vi "simx Get Joint Position.vi"(7 "operationMode":i32, 8 "error in (no error)":errorcluster, 9 "position":sgl, 10 "jointHandle":i32, 11 "clientID":i32) -> (0 "error out":errorcluster, 1 "position out":sgl, 3 "function return":i32)   [LabVIEW 2019, in "PXL_V-REP.lvlib"]
doc: "EXTAPI_DLLEXPORT simxInt simxGetJointPosition(simxInt clientID,simxInt jointHandle,simxFloat* position,simxInt operationMode);"
uses:
  PXL_V-REP.lvlib
  <userlib>/V-REP/remoteApi.dll
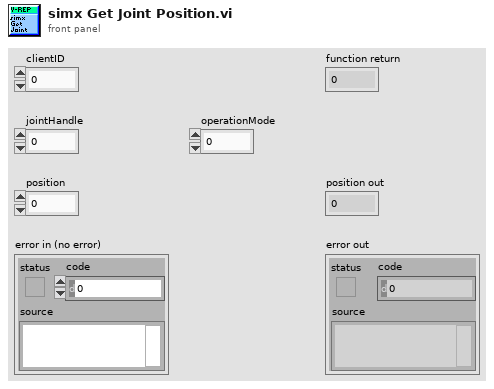
[diagram p1: front panel]
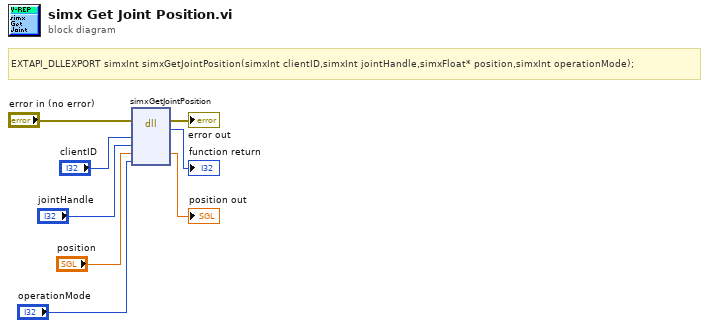
[diagram p0: block diagram]
diagram:
  # "EXTAPI_DLLEXPORT simxInt simxGetJointPosition(simxInt clientID,simxInt jointHandle,simxFloat* position,simxInt operationMode);"
  n1 = dll-call lib="C:/Program Files (x86)/National Instruments/LabVIEW 2019/user.lib/V-REP/remoteApi.*" fn="simxGetJointPosition"(error in="error in (no error)", "clientID"="clientID", "jointHandle"="jointHandle", "position"="position", "operationMode"="operationMode") -> (error out=→"error out":errorcluster, →"function return":i32, "position"=→"position out":sgl)  [unwired: 5 in, 1 out]
